vi "FromRepo.vi"(8 "error in":errorcluster, 9 "from repo cluster":T2, 10 "repository in":refnum<class "NISE_CEF_Repository.lvclass">, 11 "node in":refnum<class "Targets.lvclass">) -> (0 "error out":errorcluster, 2 "repository out":refnum<class "NISE_CEF_Repository.lvclass">, 3 "node":T1)   [LabVIEW 2019, in "Targets.lvclass"]
doc: "Grabs information from the Repo and stores it in the nodes."
uses:
  Targets.lvclass
  <vilib>/NI/Configuration Framework/Repository/NISE_CEF_Repository.lvclass
  <vilib>/NI/Configuration Framework/Node/FromRepoCluster.ctl
  <vilib>/NI/Configuration Framework/Node/NodeRef.ctl
  <vilib>/NI/Configuration Framework/Node/NISE_CEF_Node.lvclass
  CustomDeviceRepo/CustomDeviceRepo.lvclass
  C:/Program Files (x86)/National Instruments/LabVIEW 2019/vi.lib/NI/Configuration Framework/Repository/NISE_CEF_Repository.lvclass
  CustomDeviceRepo/CustomDeviceRepo.lvclass/CustomDeviceRepo.ctl
  Targets.lvclass/Targets.ctl
  CustomDeviceRepo/Read Supported Targets Properties.vi
  Write Section Name.vi
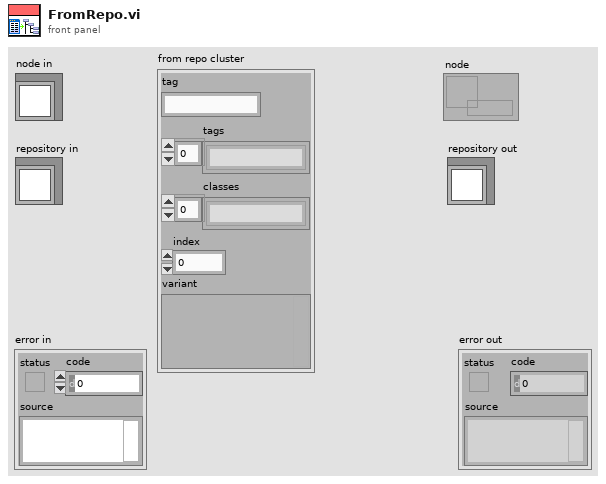
[diagram p1: front panel]
types:
  T1 = typedef "NISE_CEF_Node.lvclass/NodeRef.ctl" = refnum<data-value>
  T2 = typedef "NISE_CEF_Node.lvclass/FromRepoCluster.ctl" = cluster{"tag":string, "tags":string[], "classes":string[], "index":i32, "variant":variant}
  T3 = typedef "Source Distribution for Custom Device VI.ctl" = cluster{"Source":T4, "Real Time System Destination":string, "Supported Target":T5}[]
  T4 = typedef "Path Cluster.ctl" = cluster{"Path":path, "Path Type":enum16{"Absolute", "To Base", "To Common Doc Dir", "To Application Data Dir"}}
  T5 = typedef "Target.ctl" = enum16{"All", "Pharlap", "VxWorks", "Windows", "Linux_32_ARM", "Linux_x64", "PharlapWindows", "PharlapVxWorks", "VxWorksWindows"}
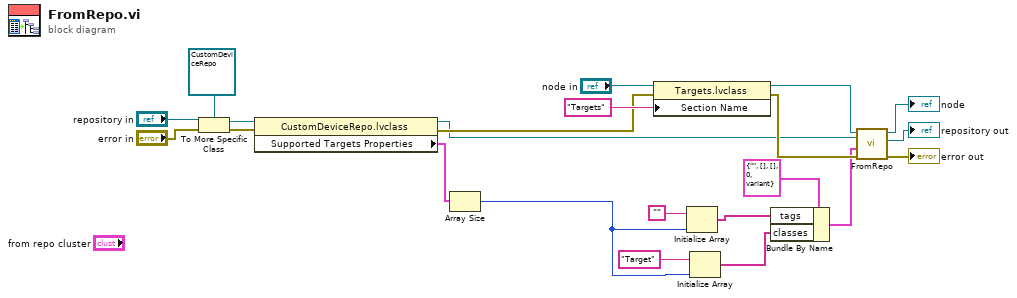
[diagram p0: block diagram]
diagram:
  n1 = To More Specific Class(target class=refnum<class "CustomDeviceRepo.lvclass"> refnum ("CustomDeviceRepo.lvclass"), reference="repository in", error in="error in") -> (specific class reference=w12:refnum<class "CustomDeviceRepo.lvclass">, error out=w11:errorcluster)
  n2 = property class="CustomDeviceRepo.lvclass"(reference=w12, error in=w11) -> (reference out=w9:refnum<class "CustomDeviceRepo.lvclass">, error out=w10:errorcluster, "Supported Targets Properties"=w7:T3)
  n3 = Array Size(array=w7) -> (size(s)=w4:i32)
  n4 = property class="Targets.lvclass"(reference="node in", error in=w10, "Section Name"="Targets") -> (reference out=w14:refnum<class "Targets.lvclass">, error out=w13:errorcluster)
  n5 = Initialize Array("", w4) -> (w3:string[])
  n6 = Initialize Array("Target", w4) -> (w2:string[])
  n7 = Bundle By Name(cluster=T2 {"tag"="", "tags"=[], "classes"=[], "index"=0, "variant"=variant} ("from repo cluster"), "tags"=w3, "classes"=w2) -> (w1:T2)
  n8 = call-parent "FromRepo.vi"("error in"=w13, "from repo cluster"=w1, "repository in"=w9, "node in"=w14) -> ("error out"=→"error out":errorcluster, "repository out"=→"repository out":refnum<class "NISE_CEF_Repository.lvclass">, "node"=→"node":T1)  [unwired: 5 in]
